vi "系统设置.vi"() -> ()   [LabVIEW 2016]
panel:
  in  "运维调试单选按钮":enum32{"营养盐", "CodMn", "总磷总氮", "多参数", "其他"}(xcontrol)
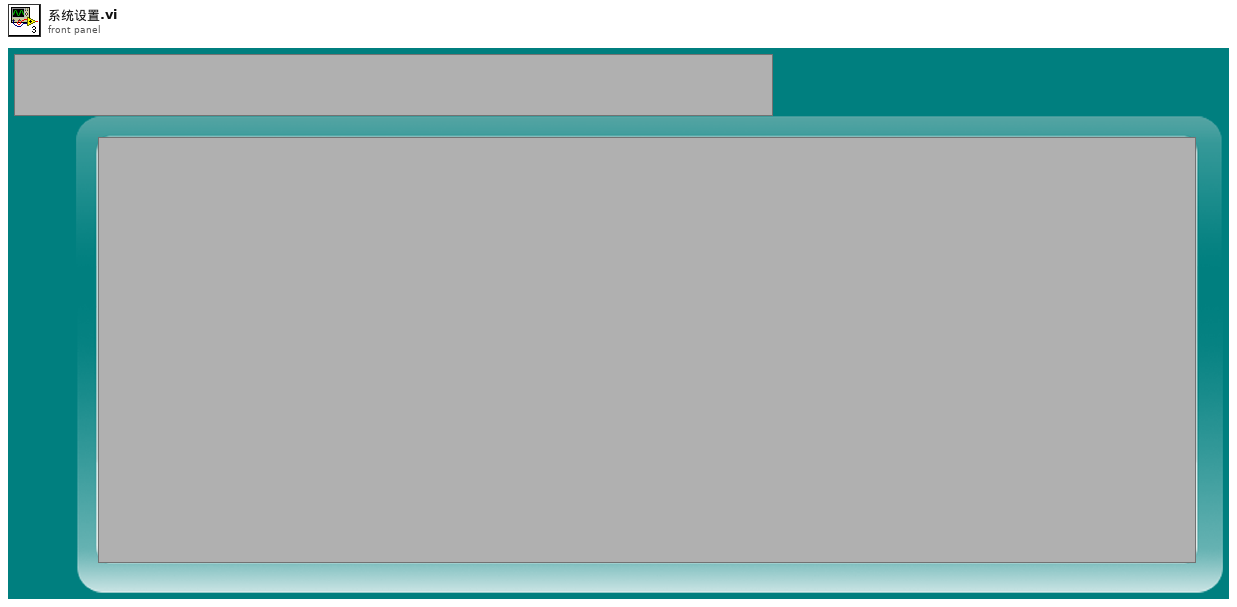
[diagram p1: front panel]
types:
  T1 = enum32{"Bad", "Idle", "Run top level", "Running"}
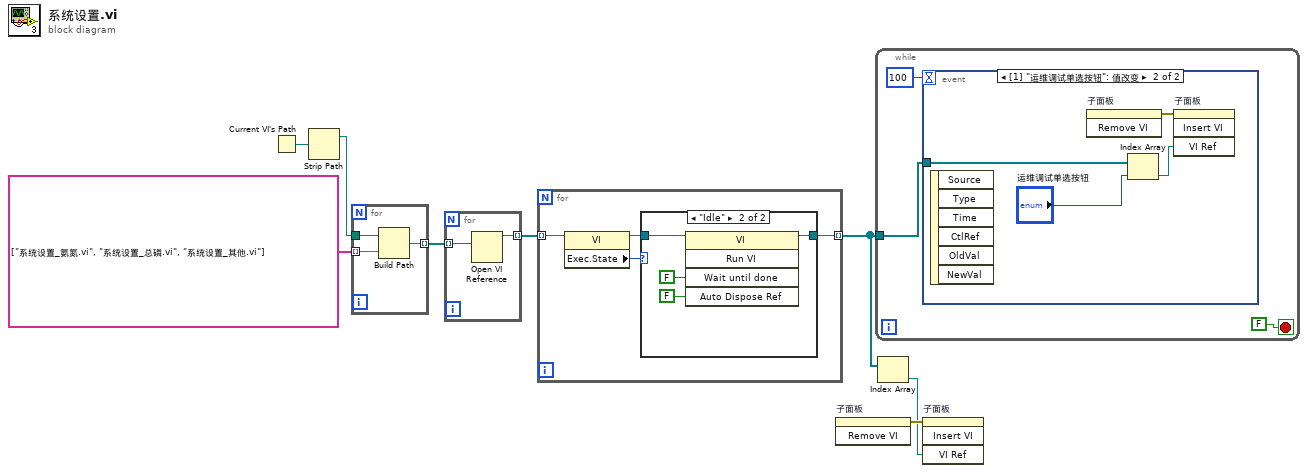
[diagram p0: block diagram]
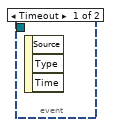
[diagram p3: hidden frame]
diagram:
  n1 = Current VI's Path() -> (path=w8:path)
  n2 = Strip Path(path=w8) -> (stripped path=w7:path)  [unwired: 1 out]
  n3 = for {
    tunnel: w7 -> [w11]
    tunnel: string[] ["系统设置_氨氮.vi", "系统设置_总磷.vi", "系统设置_其他.vi"] -> [w10] mode=indexing
    tunnel: [w9] -> w5 mode=indexing
    n4 = Build Path(base path=w11, name or relative path=w10) -> (appended path=w9:path)
  }
  n5 = for {
    tunnel: w5 -> [w13] mode=indexing
    tunnel: [w12] -> w2 mode=indexing
    n6 = Open VI Reference(vi path=w13) -> (vi reference=w12:refnum<vi>)  [unwired: 5 in, 1 out]
  }
  n7 = for {
    tunnel: w2 -> [w17] mode=indexing
    tunnel: [w14] -> w4 mode=indexing
    n8 = property class="VI"(reference=w17) -> (reference out=w15:refnum<vi>, "Exec.State"=w16:T1)  [unwired: 1 in, 1 out]
    n9 = case shown="\"Idle\"" w16 {
      tunnel: w15 -> [w18 w20]
      tunnel: [w18 w19] -> w14
      frame "Bad", Default {
      }
      frame "Idle" {
        n10 = invoke class="VI" method="Run VI"(reference=w20, "Wait until done"=FALSE ("结束前等待"), "Auto Dispose Ref"=FALSE ("自动销毁引用")) -> (reference out=w19:refnum<vi>)  [unwired: 2 in, 4 out]
      }
    }
  }
  n11 = invoke on="子面板" class="SubPnl" method="Remove VI"() -> (error out=w3:errorcluster)  [unwired: 3 in, 2 out]
  n12 = while {
    tunnel: w4 -> [w24]
    stop <- FALSE stop-if-true
    n13 = event shown="[1] \"运维调试单选按钮\": 值改变" {
      selector: _ -> [_ _]
      dyn-events: _ -> [_ _]
      timeout: 100 -> [_ _]
      tunnel: w24 -> [_ w28]
      event Timeout {
        n14 = event-data() -> ()  [unwired: 1 in, 3 out]
      }
      event "运维调试单选按钮": Value Change {
        n15 = event-data() -> ()  [unwired: 1 in, 6 out]
        n16 = invoke on="子面板" class="SubPnl" method="Remove VI"() -> (error out=w29:errorcluster)  [unwired: 3 in, 2 out]
        n17 = Index Array(array=w28, index="运维调试单选按钮") -> (element=w26:refnum<vi>)
        n18 = invoke on="子面板" class="SubPnl" method="Insert VI"(error in=w29, "VI Ref"=w26) -> ()  [unwired: 2 in, 4 out]
      }
    }
  }
  n19 = Index Array(array=w4) -> (element=w1:refnum<vi>)  [unwired: 1 in]
  n20 = invoke on="子面板" class="SubPnl" method="Insert VI"(error in=w3, "VI Ref"=w1) -> ()  [unwired: 2 in, 4 out]
